vi "Send Lookup Devices by Type.vi"(7 "Message Priority (Normal)":T1=enum."Normal", 8 "error in (no error)":errorcluster, 10 "Hardware Type":string, 11 "Message Enqueuer":refnum<class "Message Enqueuer.lvclass">) -> (0 "error out":errorcluster, 2 "Matching Devices":string[](array[string]), 3 "Message Enqueuer out":refnum<class "Message Enqueuer.lvclass">)   [LabVIEW 2015, in "Lookup Devices by Type Msg.lvclass"]
doc: "This VI sends the message to an actor."
uses:
  Lookup Devices by Type Msg.lvclass
  <vilib>/ActorFramework/Message Enqueuer/Message Enqueuer.lvclass
  <vilib>/ActorFramework/Message Enqueuer/Message Priority.ctl
  Lookup Devices by Type Msg.lvclass/Lookup Devices by Type Msg.ctl
  <vilib>/ActorFramework/Reply Msg/Reply Msg.lvclass/Reply Msg.ctl
  <vilib>/ActorFramework/Message Enqueuer/Message Enqueuer.lvclass/Message Enqueuer.ctl
  <vilib>/ActorFramework/Message Enqueuer/Enqueue.vi
  <vilib>/ActorFramework/Message Priority Queue/Priority Enqueue.vi
  <vilib>/ActorFramework/Reply Msg/Reply Msg.lvclass
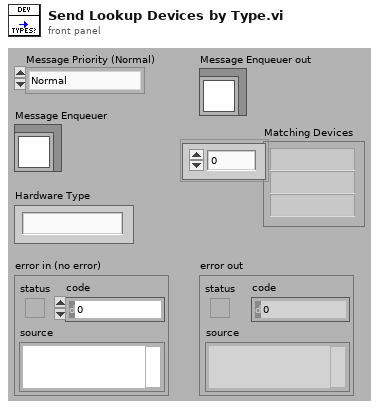
[diagram p1: front panel]
types:
  T1 = typedef "Actor Framework.lvlib/Message Enqueuer.lvclass/Message Priority.ctl" = enum16{"Low", "Normal", "High"}
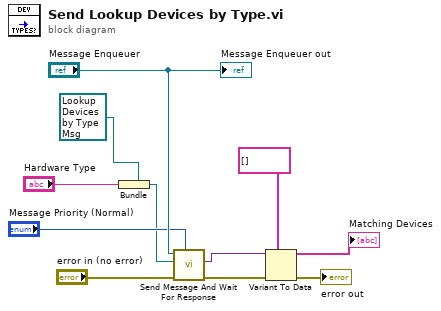
[diagram p0: block diagram]
diagram:
  n1 = Bundle(cluster=refnum<class "Lookup Devices by Type Msg.lvclass"> refnum ("Object"), "Hardware Type") -> (w6:refnum<class "Lookup Devices by Type Msg.lvclass">)
  n2 = call <vilib>:"Send Message And Wait For Response.vi"("Message Priority (Normal)"="Message Priority (Normal)", "error in (no error)"="error in (no error)", "Original Message"=w6, "Message Enqueuer in"="Message Enqueuer") -> ("error out"=w5:errorcluster, "Reply"=w4:variant)  [unwired: 4 in, 2 out]
  n3 = Variant To Data(error in=w5, type=string[] [] ("Matching Devices"), Variant=w4) -> (data=→"Matching Devices":string[], error out=→"error out":errorcluster)
  "Message Enqueuer out" <- "Message Enqueuer"
